vi "Request Task Remove.vi"(8 "error in (no error)":errorcluster, 9 "Task":refnum<class "Task.lvclass">, 10 "index":i32, 11 "Comm Interface in":refnum<class "Comm Interface.lvclass">) -> (0 "error out":errorcluster, 3 "Comm Interface out":refnum<class "Comm Interface.lvclass">)   [LabVIEW 2017, in "Comm Interface.lvlib" / "Comm Interface.lvclass"]
uses:
  Comm Interface.lvclass
  Task Interface/Task/Task.lvclass
  Message Interface/Command/Command.lvclass
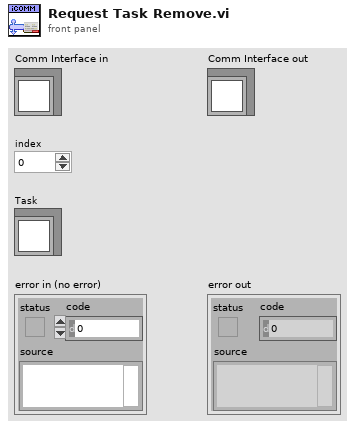
[diagram p1: front panel]
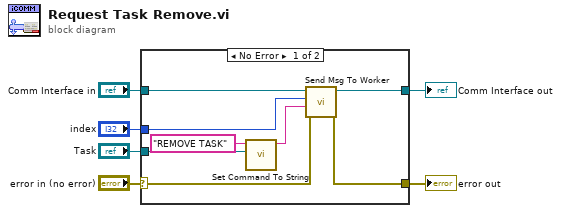
[diagram p0: block diagram]
diagram:
  n1 = case shown="No Error" "error in (no error)" {
    selector: "error in (no error)" -> [w9 w16]
    tunnel: [w8 w16] -> w5
    tunnel: [w12 w15] -> w3
    tunnel: "Comm Interface in" -> [w13 w15]
    tunnel: "index" -> [w10 _]
    tunnel: "Task" -> [w7 _]
    frame No Error {
      n2 = call "Set Command To String.vi"("Arguments"=w7, "Command"="REMOVE TASK") -> ("data string"=w11:string)  [unwired: 9 in]
      n3 = call "Send Msg To Worker.vi"("error in (no error)"=w9, "Message"=w11, "index"=w10, "Comm Interface in"=w13) -> ("error out"=w8:errorcluster, "Comm Interface out"=w12:refnum<class "Comm Interface.lvclass">)  [unwired: 6 in]
    }
    frame Error {
    }
  }
  "error out" <- w5
  "Comm Interface out" <- w3
